vi "Builder-Create Installer.vi"(0 "Exe Path":path, 5 "Product Name":string, 11 "error in (no error)":errorcluster) -> (8 "standard error":string, 15 "error out":errorcluster)   [LabVIEW 2020]
panel:
  out "standard output":string
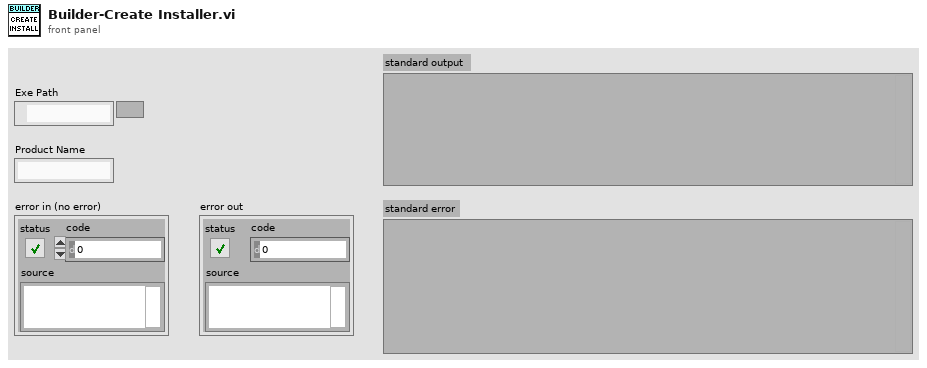
[diagram p1: front panel]
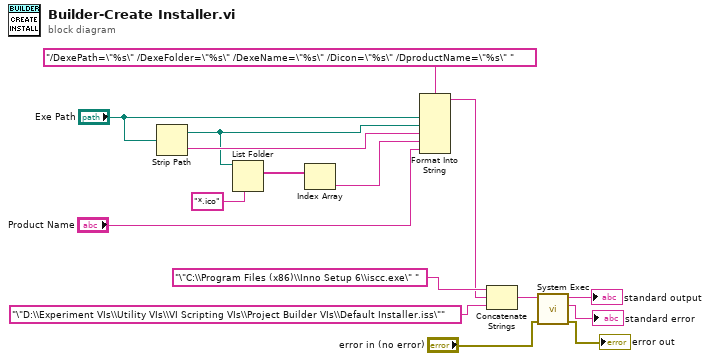
[diagram p0: block diagram]
diagram:
  n1 = Strip Path(path="Exe Path") -> (stripped path=w1:path, name=w8:string)
  n2 = List Folder(path=w1, pattern="*.ico") -> (filenames=w4:string[])  [unwired: 2 in, 3 out]
  n3 = Index Array(array=w4) -> (element=w3:string)  [unwired: 1 in]
  n4 = Format Into String(format string="/DexePath=\"%s\" /DexeFolder=\"%s\" /DexeName=\"%s\" /Dicon=\"%s\" /DproductName=\"%s\" ", "Exe Path", w1, w8, w3, "Product Name") -> (resulting string=w12:string)  [unwired: 2 in, 1 out]
  n5 = Concatenate Strings("\"C:\\Program Files (x86)\\Inno Setup 6\\iscc.exe\" " ("command line"), w12, "\"D:\\Experiment VIs\\Utility VIs\\VI Scripting VIs\\Project Builder VIs\\Default Installer.iss\"" ("command line")) -> (w15:string)
  n6 = call <vilib>:"System Exec.vi"("error in (no error)"="error in (no error)", "command line"=w15) -> ("error out"=→"error out":errorcluster, "standard error"=→"standard error":string, "standard output"=→"standard output":string)  [unwired: 6 in, 1 out]
